vi "Get.vi"(0 "object in":refnum<class "Game Board.lvclass">, 5 "error in (no error)":errorcluster) -> (16 "Game Board":u32[][](array[colorbox]), 19 "error out":errorcluster)   [LabVIEW 2021, in "Game Board.lvclass"]
uses:
  Game Board.lvclass
  Game Board.lvclass/Game Board.ctl
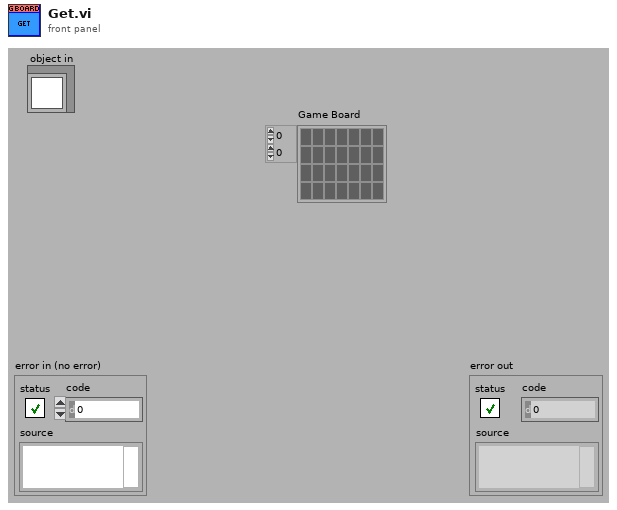
[diagram p1: front panel]
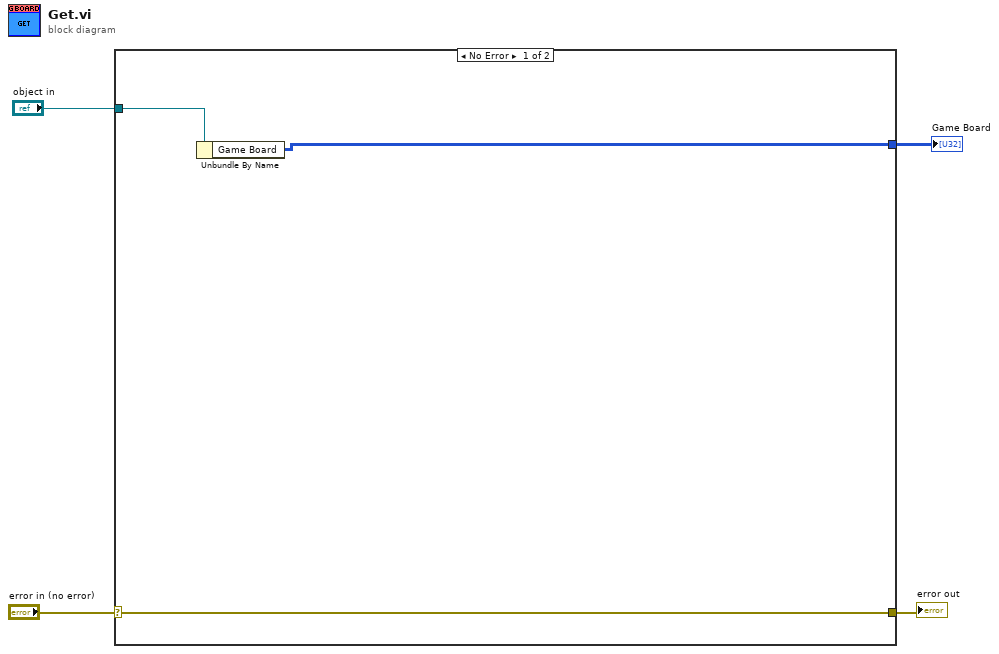
[diagram p0: block diagram]
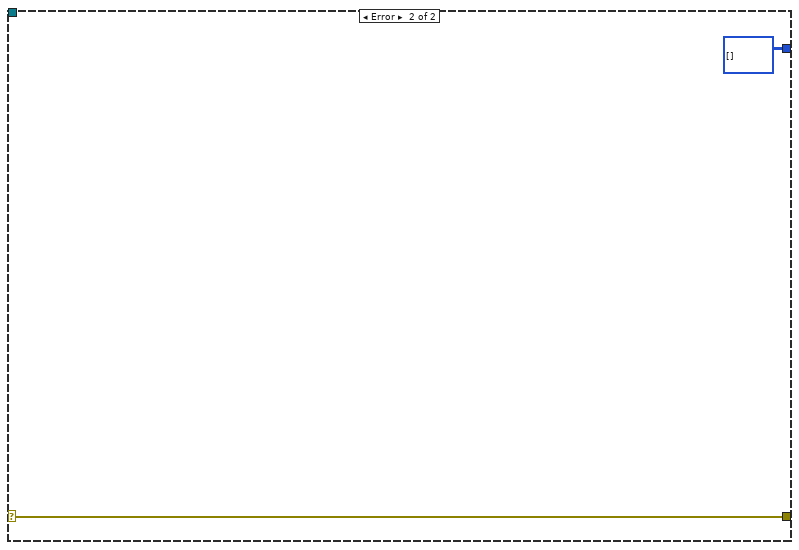
[diagram p2: hidden frame]
diagram:
  n1 = case shown="No Error" "error in (no error)" {
    selector: "error in (no error)" -> [w7 w9]
    tunnel: [w7 w9] -> w3
    tunnel: "object in" -> [w6 _]
    tunnel: [w5 u32[][] [] ("Game Board")] -> w1
    frame No Error {
      n2 = Unbundle By Name(w6) -> ("Game Board"=w5:u32[][])
    }
    frame Error {
    }
  }
  "error out" <- w3
  "Game Board" <- w1
